vi "deleteTuplaEnDBProducto.vi"(8 "error in":errorcluster, 11 "claseProducto in":refnum<class "claseProducto.lvclass">) -> (0 "error out":errorcluster, 3 "claseProducto out":refnum<class "claseProducto.lvclass">)   [LabVIEW 2014, in "claseProducto.lvclass"]
uses:
  claseProducto.lvclass
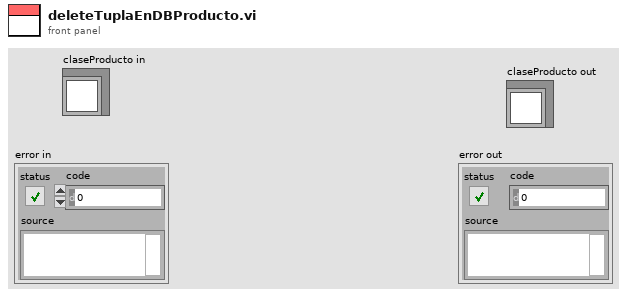
[diagram p1: front panel]
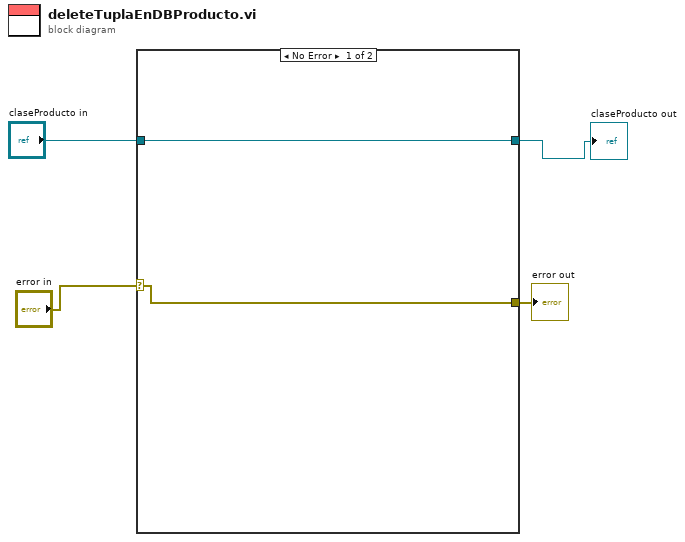
[diagram p0: block diagram]
diagram:
  n1 = case shown="No Error" "error in" {
    selector: "error in" -> [w6 w7]
    tunnel: "claseProducto in" -> [w5 w8]
    tunnel: [w6 w7] -> w2
    tunnel: [w5 w8] -> w1
    frame No Error {
    }
    frame Error {
    }
  }
  "claseProducto out" <- w1
  "error out" <- w2
